vi "Digital Output.vi"(8 "error in":errorcluster, 11 "DAQmx OutPut Setting":T1) -> (0 "error out":errorcluster, 1 "Exit":bool)   [LabVIEW 2015]
uses:
  <vilib>/DAQmx/write.llb/DAQmx Write (Digital 2D Bool NChan 1Samp NLine).vi
  <vilib>/DAQmx/write.llb/DAQmx Write (Digital 1D Bool 1Chan 1Samp).vi
  <vilib>/DAQmx/create/channels.llb/DAQmx Create Channel (DO-Digital Output).vi
  Galobal variable_TI.vi
  <vilib>/DAQmx/miscellaneous.llb/DAQmx Fill In Error Info.vi
panel:
  out "error out 2":errorcluster
  out "array":tag[](array[tag])
  out "*(type *) &x":tag
  out "Digital Output":bool[](array[boolean])
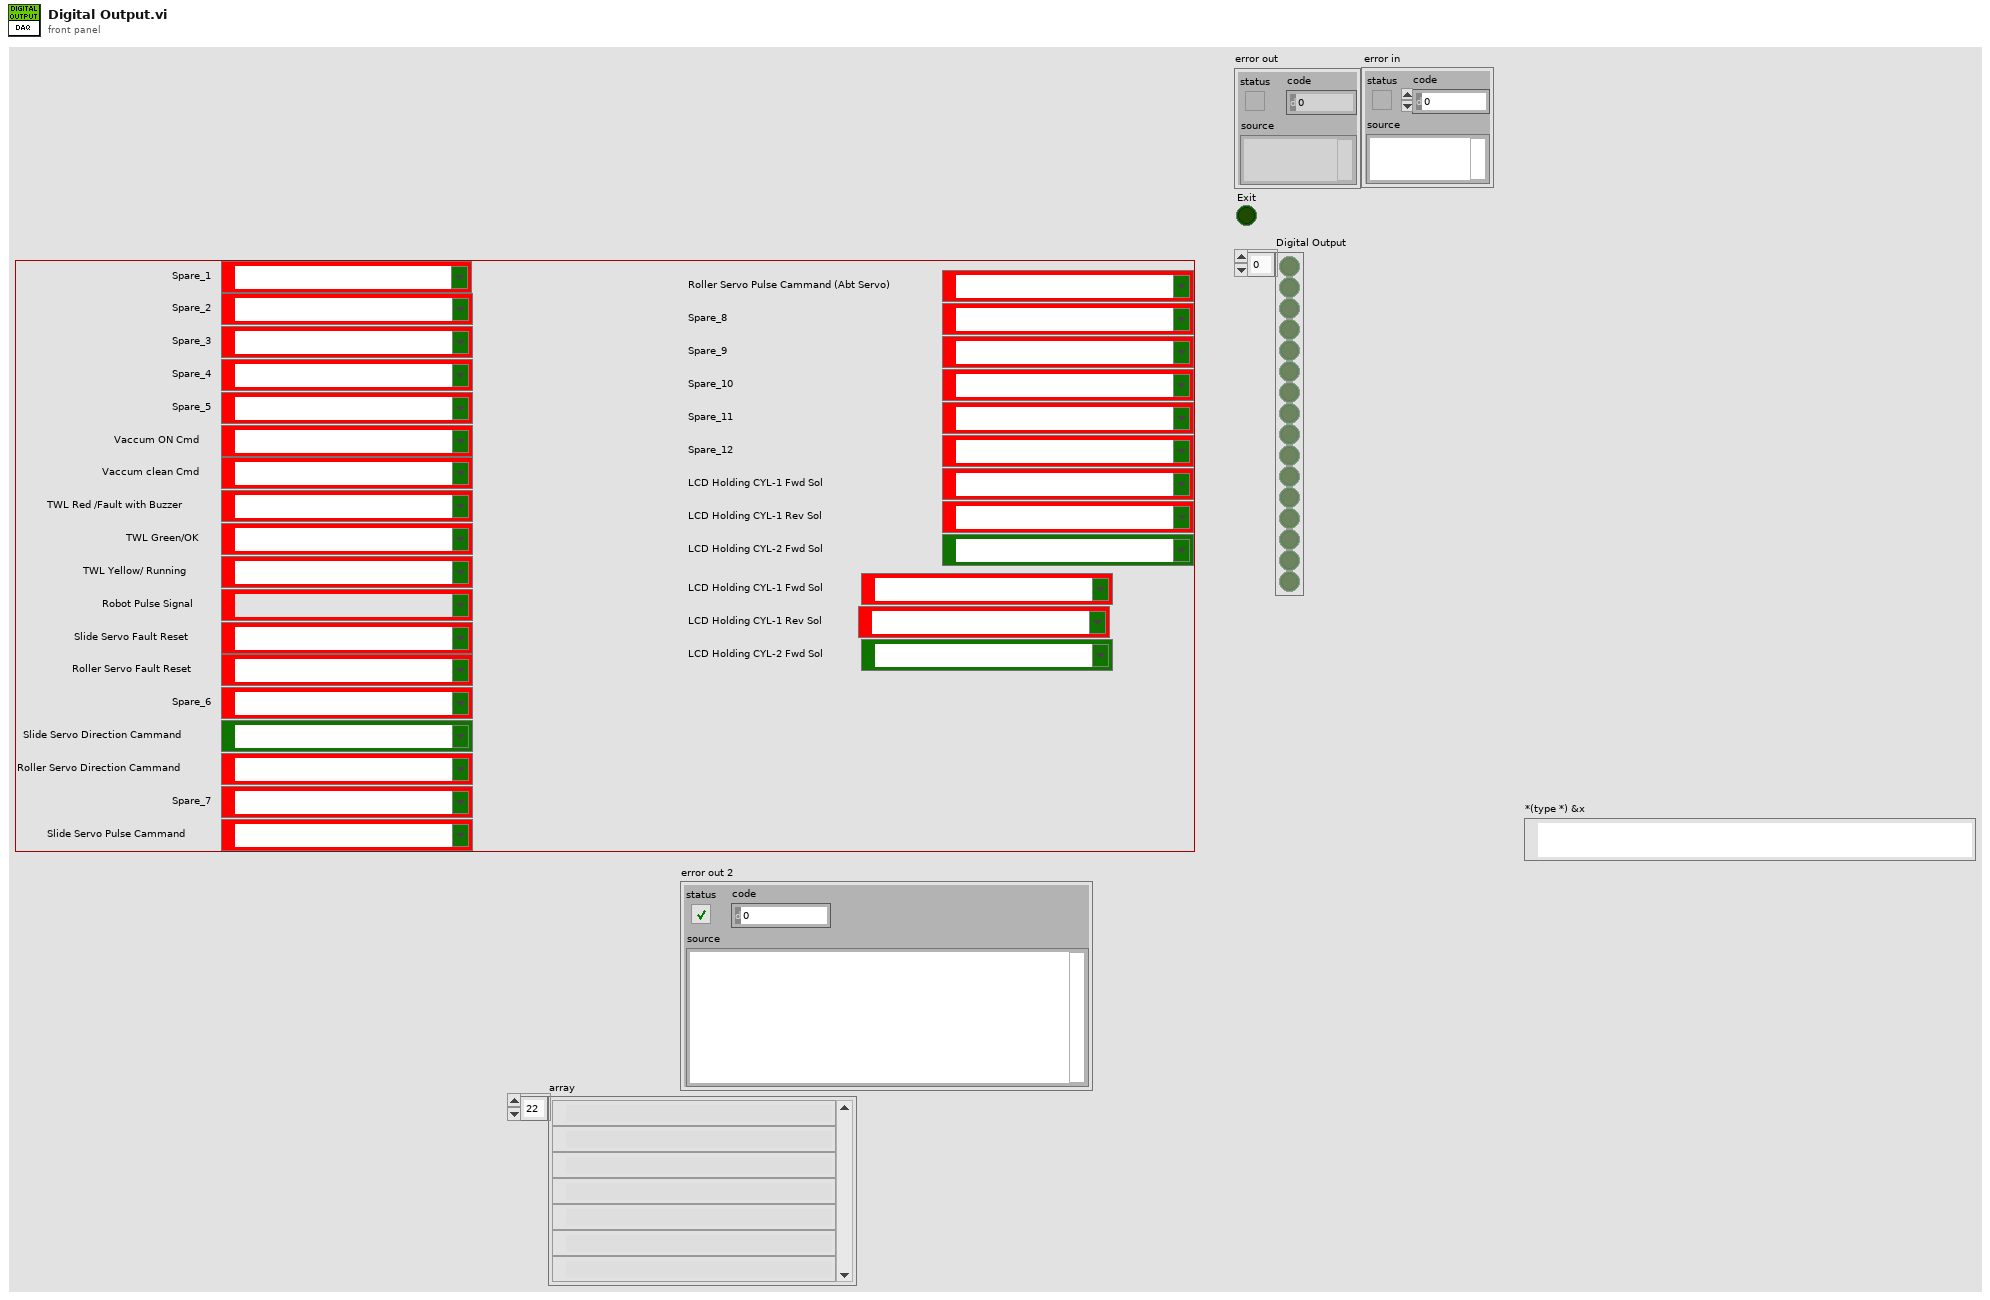
[diagram p1: front panel]
types:
  T1 = cluster{"DAQmx OutPut_00":tag, "DAQmx OutPut_01":tag, "DAQmx OutPut_02":tag, "DAQmx OutPut_03":tag, "DAQmx OutPut_04":tag, "DAQmx OutPut_05":tag, "DAQmx OutPut_06":tag, "DAQmx OutPut_07":tag, "DAQmx OutPut_08":tag, "DAQmx OutPut_09":tag, "DAQmx OutPut_10":tag, "DAQmx OutPut_11":tag, "DAQmx OutPut_12":tag, "DAQmx OutPut_13":tag, "DAQmx OutPut_14":tag, "DAQmx OutPut_15":tag, "DAQmx OutPut_16":tag, "DAQmx OutPut_17":tag, "DAQmx OutPut_18":tag, "DAQmx OutPut_19":tag, "DAQmx OutPut_20":tag, "DAQmx OutPut_21":tag, "DAQmx OutPut_22":tag, "DAQmx OutPut_23":tag, "DAQmx OutPut_12 2":tag, "DAQmx OutPut_13 2":tag, "DAQmx OutPut_14 2":tag, "DAQmx OutPut_12 3":tag, "DAQmx OutPut_13 3":tag, "DAQmx OutPut_14 3":tag}
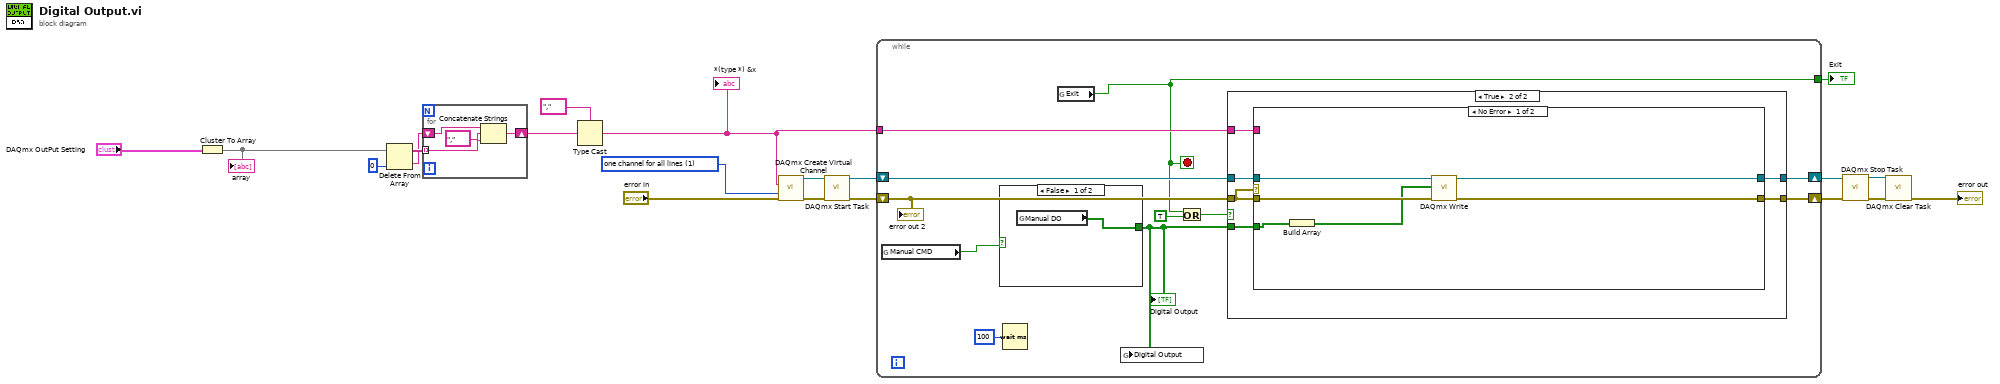
[diagram p0: block diagram]
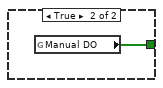
[diagram p2: hidden frame]
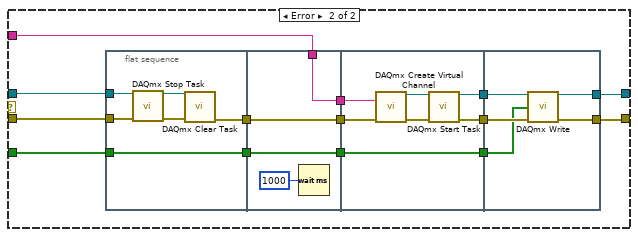
[diagram p4: hidden frame]
diagram:
  w4 = 1 items=["one channel for each line", "one channel for all lines"] ("line grouping")
  n1 = Cluster To Array(cluster="DAQmx OutPut Setting") -> (array=w2:tag[])
  "array" <- w2
  n2 = Delete From Array(array=w2, index=0) -> (deleted portion=w7:tag, array with subset deleted=w9:tag[])  [unwired: 1 in]
  n3 = for {
    tunnel: w9 -> [w23] mode=indexing
    shift-right: [w21] -> w5
    shift-left: w7 -> [w24]
    n4 = Concatenate Strings(w24, tag "," ("1."), w23) -> (w21:string)
  }
  n5 = Type Cast(type=tag "," ("1."), x=w5) -> (*(type *) &x=w3:tag)
  "*(type *) &x" <- w3
  n6 = call-poly <vilib>:"DAQmx Create Virtual Channel.vi"("lines"=w3, "line grouping"=w4, "error in"="error in") -> ("task out"=w20:refnum<k21>, "error out"=w19:errorcluster)  [unwired: 2 in, 9 out]
  n7 = call <vilib>:"DAQmx Start Task.vi"("task/channels in"=w20, "error in"=w19) -> ("task out"=w16:refnum<k21>, "error out"=w15:errorcluster)  [unwired: 12 out]
  n8 = while {
    shift-right: [w33] -> w13
    shift-left: w15 -> [w32]
    shift-right: [w34] -> w14
    shift-left: w16 -> [w35]
    tunnel: w3 -> [w31]
    tunnel: [w28] -> w10
    stop <- w28 stop-if-true
    n9 = global read "Galobal variable_TI.vi" "Manual CMD"() -> (w27:bool)
    n10 = case shown="False" w27 {
      tunnel: [w36 w37] -> w26
      frame False {
        n11 = global read "Galobal variable_TI.vi" "Manual DO"() -> (w36:bool[])
      }
      frame True {
        n12 = global read "Galobal variable_TI.vi" "Manual DO"() -> (w37:bool[])
      }
    }
    "Digital Output" <- w26
    n13 = Wait (ms)(milliseconds to wait=u32 100) -> ()  [unwired: 1 out]
    n14 = global read "Galobal variable_TI.vi" "Exit"() -> (w28:bool)
    n15 = global write "Galobal variable_TI.vi" "Digital Output"(w26) -> ()
    n16 = Or(x=w28, y=TRUE) -> (x .or. y?=w30:bool)
    n17 = case shown="True" w30 {
      tunnel: w35 -> [w39 w45]
      tunnel: [w39 w44] -> w34
      tunnel: [w38 w43] -> w33
      tunnel: w32 -> [w38 w42]
      tunnel: w31 -> [_ w41]
      tunnel: w26 -> [_ w40]
      frame False {
      }
      frame True {
        n18 = case shown="No Error" w42 {
          tunnel: w45 -> [w51 w65]
          tunnel: w42 -> [w50 w64]
          tunnel: [w49 w62] -> w44
          tunnel: [w48 w63] -> w43
          tunnel: w41 -> [_ w58]
          tunnel: w40 -> [w47 w55]
          frame No Error {
            n19 = Build Array(w47) -> (w46:bool[][])
            n20 = call-poly <vilib>:"DAQmx Write.vi"("task/channels in"=w51, "data"=w46, "error in"=w50) -> ("task out"=w49:refnum<k21>, "error out"=w48:errorcluster)  [unwired: 1 in, 10 out]
          }
          frame Error {
            n21 = flat-sequence {
              tunnel: w65 -> [w69]
              tunnel: w64 -> [w68]
              tunnel: [w67] -> w60
              tunnel: w55 -> [w66]
              tunnel: [w66] -> w54
              tunnel: [w74] -> w61
              tunnel: w60 -> [w74]
              tunnel: [w73] -> w59
              tunnel: w58 -> [w73]
              tunnel: w54 -> [w72]
              tunnel: [w72] -> w53
              tunnel: w61 -> [w78]
              tunnel: w59 -> [w77]
              tunnel: [w80] -> w57
              tunnel: [w79] -> w56
              tunnel: w53 -> [w76]
              tunnel: [w76] -> w52
              tunnel: [w85] -> w62
              tunnel: [w86] -> w63
              tunnel: w57 -> [w87]
              tunnel: w56 -> [w84]
              tunnel: w52 -> [w83]
              frame #0 {
                n22 = call <vilib>:"DAQmx Stop Task.vi"("task/channels in"=w69, "error in"=w68) -> ("task out"=w70:refnum<k21>, "error out"=w71:errorcluster)  [unwired: 12 out]
                n23 = call <vilib>:"DAQmx Clear Task.vi"("task in"=w70, "error in"=w71) -> ("error out"=w67:errorcluster)  [unwired: 13 out]
              }
              frame #1 {
                n24 = Wait (ms)(milliseconds to wait=u32 1000) -> ()  [unwired: 1 out]
              }
              frame #2 {
                n25 = call-poly <vilib>:"DAQmx Create Virtual Channel.vi"("lines"=w77, "error in"=w78) -> ("task out"=w82:refnum<k21>, "error out"=w81:errorcluster)  [unwired: 3 in, 9 out]
                n26 = call <vilib>:"DAQmx Start Task.vi"("task/channels in"=w82, "error in"=w81) -> ("task out"=w79:refnum<k21>, "error out"=w80:errorcluster)  [unwired: 12 out]
              }
              frame #3 {
                n27 = call-poly <vilib>:"DAQmx Write.vi"("task/channels in"=w84, "data"=w83, "error in"=w87) -> ("task out"=w85:refnum<k21>, "error out"=w86:errorcluster)  [unwired: 1 in, 10 out]
              }
            }
          }
        }
      }
    }
    "error out 2" <- w32
  }
  "Exit" <- w10
  n28 = call <vilib>:"DAQmx Stop Task.vi"("task/channels in"=w14, "error in"=w13) -> ("task out"=w18:refnum<k21>, "error out"=w17:errorcluster)  [unwired: 12 out]
  n29 = call <vilib>:"DAQmx Clear Task.vi"("task in"=w18, "error in"=w17) -> ("error out"=→"error out":errorcluster)  [unwired: 13 out]
